vi "conversion_pos_in_motor.vi"(3 "error in (no error)":errorcluster caption="错误输入（无错误）", 4 "pos":dbl, 5 "OneMotion 输入":refnum<class "OneMotion.lvclass">) -> (0 "error out":errorcluster caption="错误输出", 1 "pos in motor":i32, 2 "OneMotion 输出":refnum<class "OneMotion.lvclass">)   [LabVIEW 2016, in "MotionControl_UFO_3DOF.lvlib" / "OneMotion.lvclass"]
uses:
  <userlib>/MotionControl_UFO_3DOF/OneMotion/OneMotion.lvclass
  <userlib>/MotionControl_UFO_3DOF/OneMotion/unit mode.ctl
  <userlib>/MotionControl_UFO_3DOF/OneMotion/OneMotion.lvclass/OneMotion.ctl
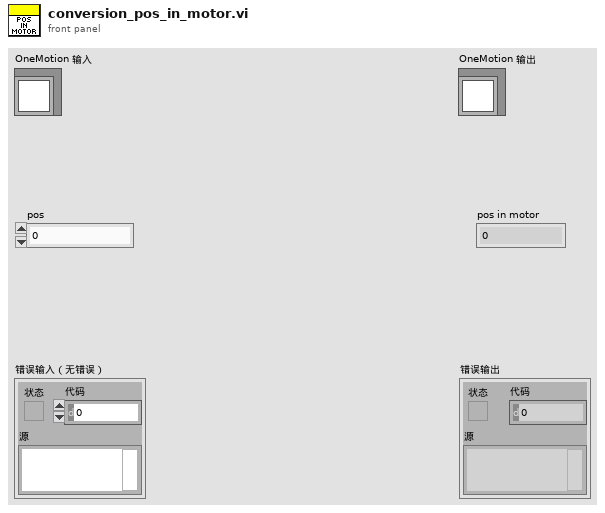
[diagram p1: front panel]
types:
  T1 = typedef "MotionControl_UFO_3DOF.lvlib/OneMotion.lvclass/unit mode.ctl" = enum16{"motor (pulse)", "linear (mm) or radial (degree)"}
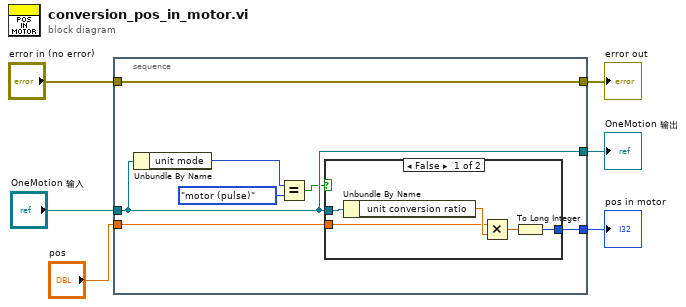
[diagram p0: block diagram]
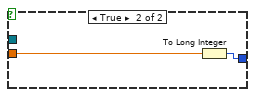
[diagram p2: hidden frame]
diagram:
  n1 = stacked-sequence {
    tunnel: [w10] -> w6
    tunnel: [w13] -> w4
    tunnel: "OneMotion 输入" -> [w13]
    tunnel: "pos" -> [w12]
    tunnel: [w11] -> w2
    tunnel: "error in (no error)" -> [w10]
    frame #0 {
      n2 = Unbundle By Name(w13) -> ("unit mode"=w8:T1)
      n3 = Equal?(x=w8, y=unit_mode."motor (pulse)" ("unit mode")) -> (x = y?=w7:bool)
      n4 = case shown="False" w7 {
        tunnel: [w14 w19] -> w11
        tunnel: w13 -> [w18 _]
        tunnel: w12 -> [w15 w20]
        frame False {
          n5 = Unbundle By Name(w18) -> ("unit conversion ratio"=w16:dbl)
          n6 = Multiply(x=w15, y=w16) -> (x*y=w17:dbl)
          n7 = To Long Integer(number=w17) -> (32bit integer=w14:i32)
        }
        frame True {
          n8 = To Long Integer(number=w20) -> (32bit integer=w19:i32)
        }
      }
    }
  }
  "error out" <- w6
  "OneMotion 输出" <- w4
  "pos in motor" <- w2
